vi "image tes.vi"(0 "ROI Descriptor (Color Classification 3)":T1={"Global Rectangle"=[0, 0, 1279, 959], "Contours"=[{"ID"=enum."External", "Type"=3, "Coordinates"=[0, 0, 1279, 959]}]} {"Contours"."Type" items=["No Selection", "Point", "Line", "Rectangle", "Oval", "Polygon", "Freehand Region", "Annulus", "Unused2", "Unused3", "Broken Line", "Freehand Line", "Rotated Rectangle"]}, 7 "error in":errorcluster) -> (20 "Classes (Color Classification 3)":string[](array[string]), 27 "error out":errorcluster)   [LabVIEW 2019]
uses:
  <vilib>/vision/Classification.llb/IMAQ Classifier Read Options.ctl
  <vilib>/vision/NI_Vision_Development_Module.lvlib
panel:
  out "Image Out":T2(plugin-control)
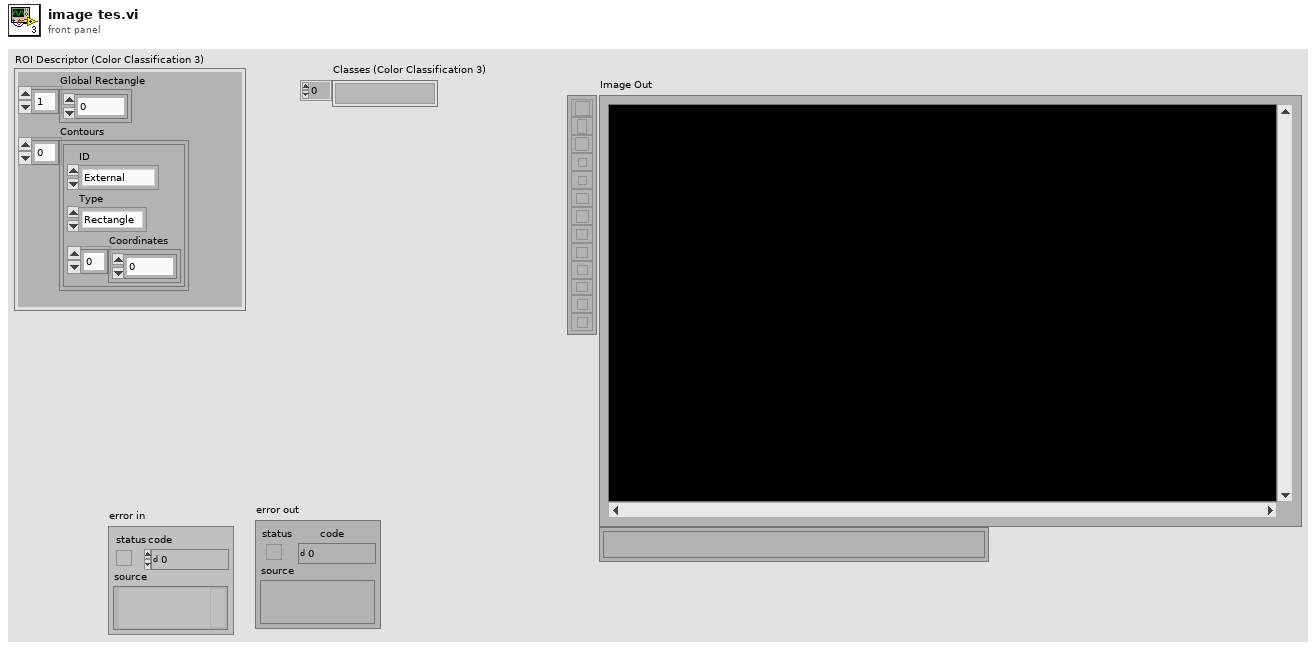
[diagram p1: front panel]
types:
  T1 = cluster{"Global Rectangle":i32[], "Contours":cluster{"ID":enum32{"External", "Internal"}, "Type":u32, "Coordinates":i32[]}[]}
  T2 = typedef "IMAQ Image.ctl" = refnum<image>
  T3 = typedef "IMAQ Classifier Read Options.ctl" = i32
  T4 = typedef "IMAQ Classifier Session.ctl" = refnum<k1>
  T5 = typedef "ROI Descriptor" = cluster{"Global Rectangle":i32[], "Contours":cluster{"ID":enum32{"External", "Internal"}, "Type":u32, "Coordinates":i32[]}[]}
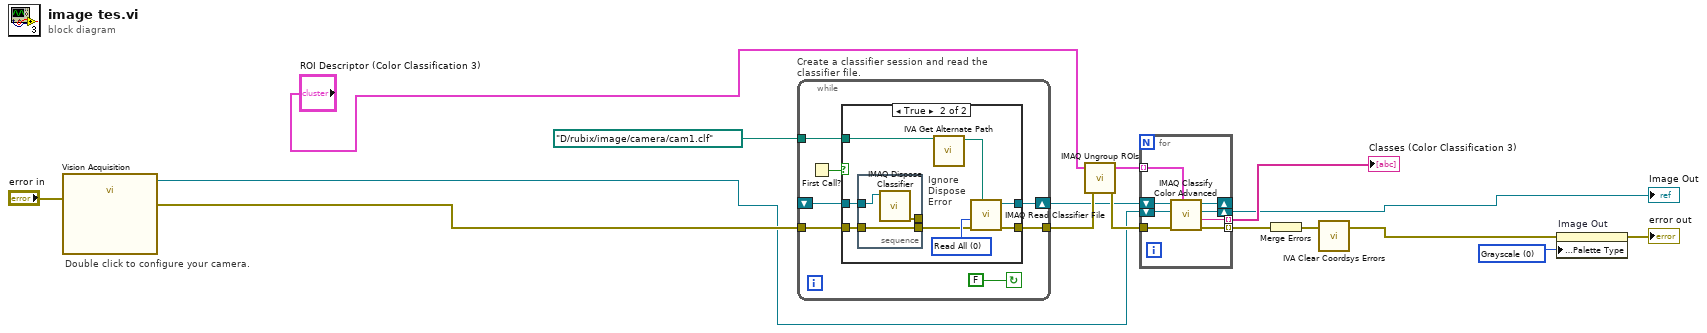
[diagram p0: block diagram]
diagram:
  w1 = u32 0 items=["Grayscale", "Binary", "Gradient", "Rainbow", "Temperature", "User Defined", "Binary 16 Bit", "Gradient 16 Bit", "Rainbow 16 Bit", "Temperature 16 Bit", "User Defined 16 Bit"] ("Palette Type")
  # "Double click to configure your camera."
  n1 = call "Vision Acquisition"("error in"="error in") -> ("Image Out"=w5:T2, "error out"=w15:errorcluster)  [unwired: 25 in]
  n2 = while "Create a classifier session and read the classifier file." {
    shift-right: [w23] -> w4
    shift-left: _ -> [w22]
    tunnel: w15 -> [w20]
    tunnel: [w19] -> w11
    tunnel: path "D:/rubix/image/camera/cam1.clf" ("File Path") -> [w18]
    stop <- FALSE continue-if-true
    n3 = First Call?() -> (First Call?: T/F=w17:bool)
    n4 = case shown="True" w17 {
      tunnel: [w25 w32] -> w23
      tunnel: w22 -> [w25 w30]
      tunnel: w20 -> [w24 w29]
      tunnel: [w24 w31] -> w19
      tunnel: w18 -> [_ w27]
      frame False {
      }
      frame True {
        w33 = T3 0 items=["Read All", "Add Samples, Do Not Change Options", "Read Options, Do Not Add Samples"] ("Read Options")
        # "Ignore Dispose Error"
        n5 = stacked-sequence {
          tunnel: w30 -> [w36]
          tunnel: w29 -> [w35]
          tunnel: [w35] -> w28
          tunnel: [w34] -> _
          frame #0 {
            n6 = call "IMAQ Dispose Classifier"("Classifier Session"=w36) -> ("error out"=w34:errorcluster)  [unwired: 1 in, 9 out]
          }
        }
        n7 = call <vilib>:"IVA Get Alternate Path.vi"("Path In"=w27) -> ("Path Out"=w26:path)  [unwired: 10 out]
        n8 = call "IMAQ Read Classifier File"("File Path"=w26, "error in (no error)"=w28, "Read Options"=w33) -> ("error out"=w31:errorcluster, "Classifier Session"=w32:T4)  [unwired: 1 in, 6 out]
      }
    }
  }
  n9 = call "IMAQ Ungroup ROIs"("error in (no error)"=w11, "ROI Descriptor"="ROI Descriptor (Color Classification 3)") -> ("error out"=w10:errorcluster, "ROI Descriptors out"=w9:T5[])  [unwired: 2 out]
  n10 = for {
    tunnel: [w44] -> w13 mode=indexing
    tunnel: [w43] -> w8 mode=indexing
    tunnel: w10 -> [w41]
    tunnel: w9 -> [w40] mode=indexing
    shift-right: [w38] -> w2
    shift-left: w5 -> [w39]
    shift-right: [w37] -> _
    shift-left: w4 -> [w42]
    n11 = call "IMAQ Classify Color Advanced"("ROI Descriptor"=w40, "error in (no error)"=w41, "Image"=w39, "Classifier Session"=w42) -> ("error out"=w43:errorcluster, "Class"=w44:string, "Image (dup)"=w38:T2, "Classifier Session (dup)"=w37:T4)  [unwired: 4 out]
  }
  "Classes (Color Classification 3)" <- w13
  "Image Out" <- w2
  n12 = Merge Errors(w8) -> (w7:errorcluster)
  n13 = call <vilib>:"IVA Clear Coordsys Errors.vi"("error in (no error)"=w7) -> ("error out"=w6:errorcluster)  [unwired: 10 in]
  n14 = property on="Image Out" class="ImageControl"(error in=w6, "Palette:Palette Type"=w1) -> (error out=→"error out":errorcluster)  [unwired: 1 in, 1 out]
